vi "getTokenElement.vi"(7 "Endpoint Element Name":string, 8 "error in (no error)":errorcluster, 10 "Token element":T1, 11 "Oauth2 in":refnum<class "Oauth2.lvclass">) -> (0 "error out":errorcluster, 1 "Value":string, 2 "Key":string, 3 "Oauth2 out":refnum<class "Oauth2.lvclass">, 4 "element found":bool)   [LabVIEW 2020, in "Oauth2.lvclass"]
uses:
  Oauth2.lvclass
  Oauth2.lvclass/Oauth2.ctl
  OAuthToken/OAuthAccessToken.lvclass
  OAuthToken/OAuth2 Token Element -- enum.ctl
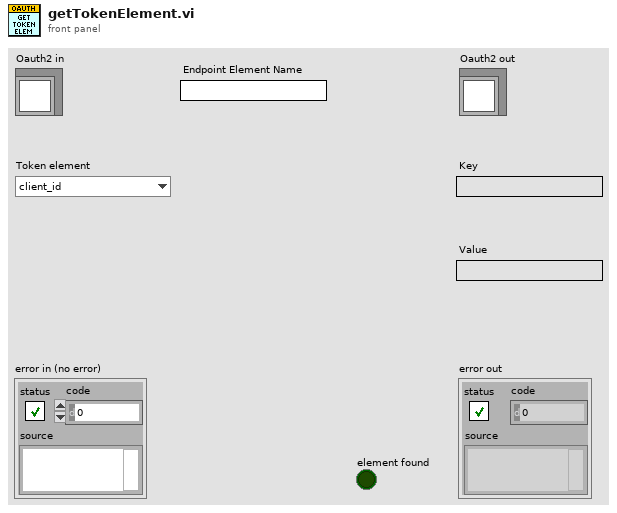
[diagram p1: front panel]
types:
  T1 = typedef "OAuthAccessToken.lvclass/OAuth2 Token Element -- enum.ctl" = enum16{"client_id", "client_secret", "response_type", "scope", "redirect_uri", "error", "error_description", "error_uri", "grant_type", "code", "access_token", "token_type", "expires_in", "username", "password", "refresh_token", "code_challenge", "code_challenge_method", "reverse_proxy_uri", "endpoint element"}
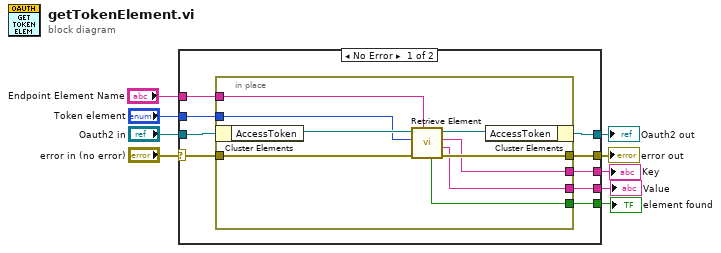
[diagram p0: block diagram]
diagram:
  n1 = case shown="No Error" "error in (no error)" {
    selector: "error in (no error)" -> [w16 w29]
    tunnel: [w15 w29] -> w8
    tunnel: [w17 w28] -> w6
    tunnel: "Oauth2 in" -> [w18 w28]
    tunnel: "Token element" -> [w14 _]
    tunnel: "Endpoint Element Name" -> [w13 _]
    tunnel: [w12 _] -> w3
    tunnel: [w11 _] -> w2
    tunnel: [w10 _] -> w1
    frame No Error {
      n2 = in-place {
        in-place-border: w16 -> [w24]
        in-place-border: [w23] -> w15
        in-place-border: w14 -> [w25]
        in-place-border: w13 -> [w27]
        in-place-border: [w21] -> w12
        in-place-border: [w20] -> w11
        in-place-border: [w19] -> w10
        n3 = in-place-cluster #1(w18) -> ("AccessToken"=w26:refnum<class "OAuthAccessToken.lvclass">)
        n4 = call "Retrieve Element.vi"("Endpoint element key"=w27, "error in (no error)"=w24, "Token element"=w25, "OAuthAccessToken in"=w26) -> ("error out"=w23:errorcluster, "Value"=w20:string, "Key"=w21:string, "OAuthAccessToken out"=w22:refnum<class "OAuthAccessToken.lvclass">, "element found"=w19:bool)  [unwired: 3 in]
        n5 = in-place-cluster #1("AccessToken"=w22) -> (w17:refnum<class "Oauth2.lvclass">)
      }
    }
    frame Error {
    }
  }
  "error out" <- w8
  "Oauth2 out" <- w6
  "Value" <- w2
  "Key" <- w3
  "element found" <- w1
